vi "__List Cloud Path.vi"(8 "error in (no error)":errorcluster, 10 "Bucket":string, 11 "Path":string) -> (0 "error out":errorcluster, 2 "Folders":string[](array[string]), 3 "Objects":T1[](array[typedef]))   [LabVIEW 2011]
doc: "This VI lists the objects that reside in an Amazon S3 bucket under the specified path.\nItems are returned in two groups: objects (files) and folders."
uses:
  __Cloud Object Info type.ctl
  vi.lib/National Instruments/LabVIEW Interface for Amazon S3/Typedefs/AMZ_S3_Storage Class.ctl
  vi.lib/National Instruments/LabVIEW Interface for Amazon S3/Typedefs/AMZ_S3_API_GET Bucket Request Parameters.ctl
  vi.lib/National Instruments/LabVIEW Interface for Amazon S3/LV Interface for Amazon S3.lvlib
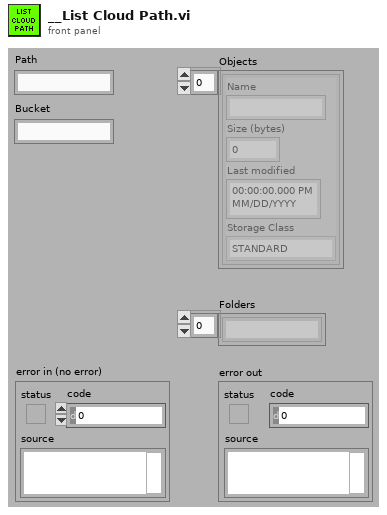
[diagram p1: front panel]
types:
  T1 = typedef "__Cloud Object Info type.ctl" = cluster{"Name":string, "Size (bytes)":u64, "Last modified":timestamp, "Storage Class":T2}
  T2 = typedef "LV Interface for Amazon S3.lvlib/AMZ_S3_Storage Class.ctl" = enum16{"STANDARD", "REDUCED_REDUNDANCY"}
  T3 = typedef "LV Interface for Amazon S3.lvlib/AMZ_S3_API_GET Bucket Request Parameters.ctl" = cluster{"delimiter":string, "marker":string, "max-keys":u16, "prefix":string}
  T4 = typedef "LV Interface for Amazon S3.lvlib/AMZ_S3_API_ListBucketResult.ctl" = cluster{"Name":string, "Prefix":string, "Marker":string, "MaxKeys":u16, "IsTruncated?":bool, "Contents":T5[], "CommonPrefixes":T7[]}
  T5 = typedef "LV Interface for Amazon S3.lvlib/AMZ_S3_API_ListBucketResult Content.ctl" = cluster{"Key":string, "LastModified":timestamp, "ETag":string, "Size":u64, "Storage Class":T2, "Owner":T6}
  T6 = typedef "LV Interface for Amazon S3.lvlib/AMZ_S3_API_Owner.ctl" = cluster{"ID":string, "DisplayName":string}
  T7 = typedef "LV Interface for Amazon S3.lvlib/AMZ_S3_API_ListBucketResult CommonPrefix.ctl" = cluster{"Prefix":string}
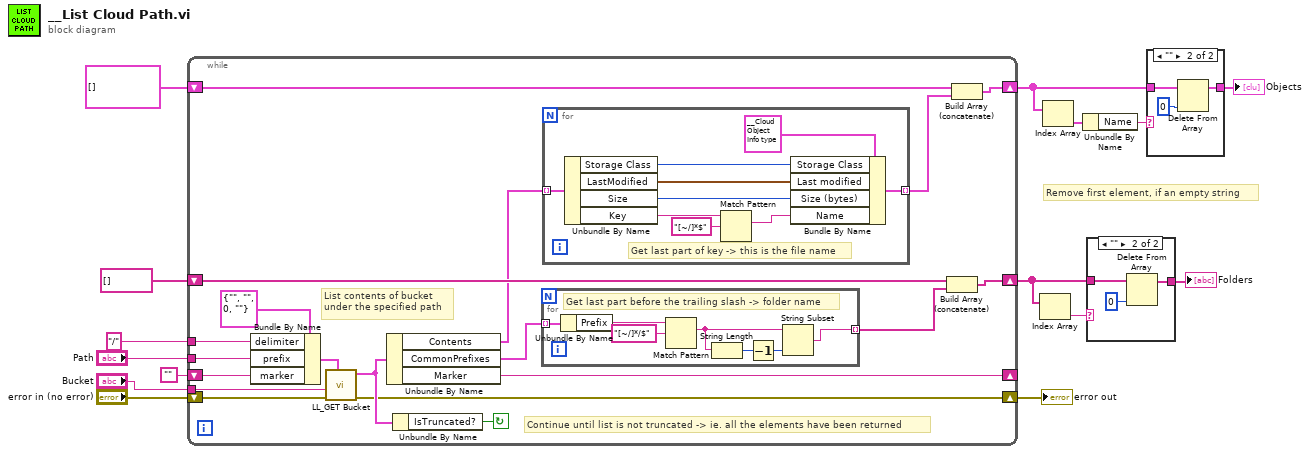
[diagram p0: block diagram]
diagram:
  # "Remove first element, if an empty string"
  n1 = while {
    tunnel: "Bucket" -> [w33]
    tunnel: "/" ("delimiter") -> [w31]
    tunnel: "Path" -> [w29]
    shift-right: [w16] -> w2
    shift-left: T1[] [] ("Array") -> [w18]
    shift-right: [w20] -> w6
    shift-left: string[] [] -> [w24]
    shift-right: [w23] -> _
    shift-left: "" -> [w26]
    shift-right: [w25] -> w10
    shift-left: "error in (no error)" -> [w34]
    stop <- w28 continue-if-true
    # "List contents of bucket\nunder the specified path"
    # "Continue until list is not truncated -> ie. all the elements have been returned"
    n2 = Bundle By Name(cluster=T3 {"delimiter"="", "marker"="", "max-keys"=0, "prefix"=""} ("GET Bucket Request Parameters"), "delimiter"=w31, "prefix"=w29, "marker"=w26) -> (w30:T3)
    n3 = call "LL_GET Bucket.vi"("GET Bucket Request Parameters"=w30, "error in (no error)"=w34, "Bucket"=w33) -> ("error out"=w25:errorcluster, "ListBucketResult"=w27:T4)  [unwired: 6 in, 1 out]
    n4 = Unbundle By Name(w27) -> ("Contents"=w19:T5[], "CommonPrefixes"=w22:T7[], "Marker"=w23:string)
    n5 = Unbundle By Name(w27) -> ("IsTruncated?"=w28:bool)
    n6 = for {
      tunnel: w22 -> [w50] mode=indexing
      tunnel: [w44] -> w21 mode=indexing
      # "Get last part before the trailing slash -> folder name"
      n7 = Unbundle By Name(w50) -> ("Prefix"=w48:string)
      n8 = Match Pattern(string=w48, regular expression="[~/]*/$") -> (match substring=w47:string)  [unwired: 1 in, 3 out]
      n9 = String Length(string=w47) -> (length=w46:i32)
      n10 = Decrement(x=w46) -> (x-1=w45:i32)
      n11 = String Subset(string=w47, length (rest)=w45) -> (substring=w44:string)  [unwired: 1 in]
    }
    n12 = for {
      tunnel: w19 -> [w43] mode=indexing
      tunnel: [w36] -> w17 mode=indexing
      # "Get last part of key -> this is the file name"
      n13 = Unbundle By Name(w43) -> ("Storage Class"=w38:T2, "LastModified"=w37:timestamp, "Size"=w39:u64, "Key"=w41:string)
      n14 = Match Pattern(string=w41, regular expression="[~/]*$") -> (match substring=w35:string)  [unwired: 1 in, 3 out]
      n15 = Bundle By Name(cluster=T1 {"Name"="", "Size (bytes)"=0, "Last modified"=timestamp(0 s since 1904-01-01), "Storage Class"=enum."STANDARD"}, "Storage Class"=w38, "Last modified"=w37, "Size (bytes)"=w39, "Name"=w35) -> (w36:T1)
    }
    n16 = Build Array (concatenate)(w24, w21) -> (w20:string[])
    n17 = Build Array (concatenate)(w18, w17) -> (w16:T1[])
  }
  "error out" <- w10
  n18 = Index Array(array=w6) -> (element=w5:string)  [unwired: 1 in]
  n19 = Index Array(array=w2) -> (element=w4:T1)  [unwired: 1 in]
  n20 = Unbundle By Name(w4) -> ("Name"=w3:string)
  n21 = case shown="\"\"" w5 {
    tunnel: [w51 w53] -> w7
    tunnel: w6 -> [w51 w52]
    frame Default {
    }
    frame "" {
      n22 = Delete From Array(array=w52, index=0) -> (array with subset deleted=w53:string[])  [unwired: 1 in, 1 out]
    }
  }
  "Folders" <- w7
  n23 = case shown="\"\"" w3 {
    tunnel: w2 -> [w55 w57]
    tunnel: [w55 w56] -> w1
    frame Default {
    }
    frame "" {
      n24 = Delete From Array(array=w57, index=0) -> (array with subset deleted=w56:T1[])  [unwired: 1 in, 1 out]
    }
  }
  "Objects" <- w1
